vi "DC Voltage Source (DAQmx) - Copy.vi"() -> ()   [LabVIEW 2009]
uses:
  <vilib>/DAQmx/create/channels.llb/DAQmx Create Channel (AO-Voltage-Basic).vi
  <vilib>/DAQmx/write.llb/DAQmx Write (Analog DBL 1Chan 1Samp).vi
panel:
  in  "Knob":dbl(knob) min=-10.0 max=10.0 step=0.2 scale=-4.0..4.0 scale format="%#.4g"
  in  "physical channels":tag
  in  "stop":bool
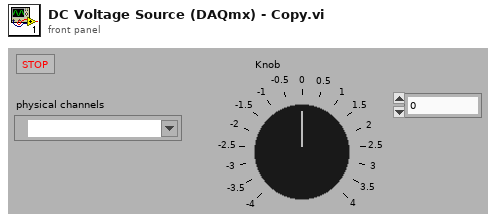
[diagram p1: front panel]
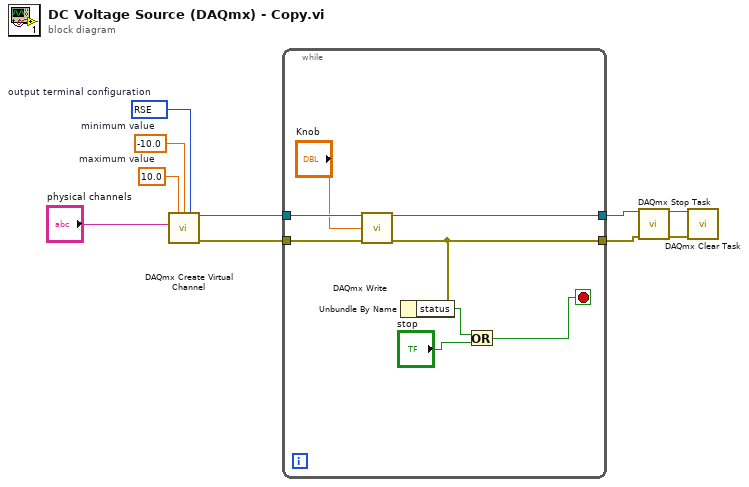
[diagram p0: block diagram]
diagram:
  w8 = 10083 items=["default"=-1, "RSE"=10083, "NRSE"=10078, "Differential"=10106, "Pseudodifferential"=12529]  # output terminal configuration
  w9 = -10.0  # minimum value
  w10 = 10.0  # maximum value
  n1 = call-poly <vilib>:"DAQmx Create Virtual Channel.vi"("maximum value"=w10, "minimum value"=w9, "output terminal configuration"=w8, "physical channels"="physical channels") -> ("task out"=w7:refnum<k21>, "error out"=w6:errorcluster)  [unwired: 5 in, 5 out]
  n2 = while {
    tunnel: w7 -> [w18]
    tunnel: w6 -> [w17]
    tunnel: [w16] -> w3
    tunnel: [w15] -> w4
    stop <- w11 stop-if-true
    n3 = call-poly <vilib>:"DAQmx Write.vi"("task/channels in"=w18, "data"="Knob", "error in"=w17) -> ("task out"=w15:refnum<k21>, "error out"=w16:errorcluster)  [unwired: 1 in, 10 out]
    n4 = Unbundle By Name(w16) -> ("status"=w13:bool)
    n5 = Or(x=w13, y="stop") -> (x .or. y?=w11:bool)
  }
  n6 = call <vilib>:"DAQmx Stop Task.vi"("task/channels in"=w4, "error in"=w3) -> ("task out"=w2:refnum<k21>, "error out"=w1:errorcluster)  [unwired: 12 in]
  n7 = call <vilib>:"DAQmx Clear Task.vi"("task in"=w2, "error in"=w1) -> ()  [unwired: 13 in, 1 out]
